vi "Get MDIF Blocks.vi"   [LabVIEW 2023, in "NI_HFNetworkAnalysis.lvlib"]
doc: "Retrieve the MDIF blocks available in memory for the referenced MDIF file."
uses:
  NI_HFNetworkAnalysis.lvlib
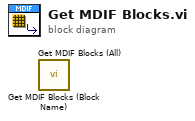
[diagram p0: block diagram]
diagram:
  n1 = call "Get MDIF Blocks (Block Name).vi"() -> ()  [unwired: 9 in, 3 out]
  n2 = call "Get MDIF Blocks (All).vi"() -> ()  [unwired: 9 in, 3 out]
